vi "UpdateReferencePoints From ResultTable.vi"(11 "MulticolumnListbox in":refnum<vi>) -> (3 "Array":string[][](array[string]))   [LabVIEW 2015]
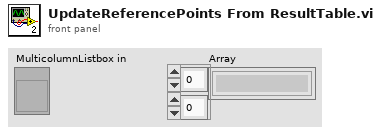
[diagram p1: front panel]
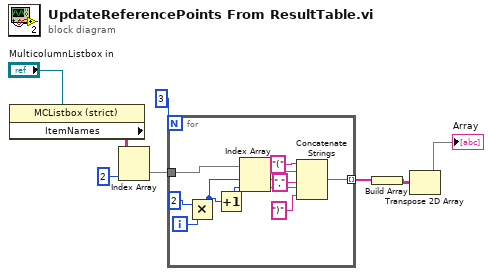
[diagram p0: block diagram]
diagram:
  n1 = property class="MCListbox (strict)"(reference="MulticolumnListbox in") -> ("ItemNames"=w2:string[][])  [unwired: 1 in, 2 out]
  n2 = Index Array(array=w2, index (col)=2 ("disabled index (col)")) -> (element=w5:string[])  [unwired: 1 in]
  n3 = for {
    N: 3 -> [_]
    tunnel: w5 -> [w19]
    tunnel: [w9] -> w6 mode=indexing
    i -> [w18]
    n4 = Multiply(x=2, y=w18) -> (x*y=w16:i32)
    n5 = Increment(x=w16) -> (x+1=w15:i32)
    n6 = Index Array(array=w19, index #1=w16, index #2=w15) -> (element #1=w14:string, element #2=w11:string)
    n7 = Concatenate Strings("(" ("string"), w14, "," ("string"), w11, ")" ("string")) -> (w9:string)
  }
  n8 = Build Array(w6) -> (w7:string[][])
  n9 = Transpose 2D Array(2D array=w7) -> (transposed array=→"Array":string[][])
